vi "Mouse Init.vi"(2 "Timeout (ms)":i32=100, 3 "FPGA VI Reference In":refnum<k20>) -> (0 "Timed out?":bool, 1 "Mouse Sensor":T1)   [LabVIEW 2012, in "Mouse IO.lvlib"]
uses:
  Mouse IO.lvlib
panel:
  # "Mouse Interface\n===\nInitialise and begin Mouse Sensor.\nReturns Mouse Sensor cluster to pass to Mouse Loop.vi\nTimeout in 100's of milliseconds."
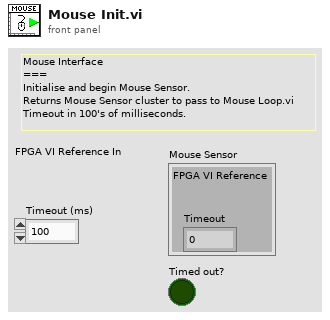
[diagram p1: front panel]
types:
  T1 = cluster{"FPGA VI Reference":refnum<k20>, "Timeout":i32}
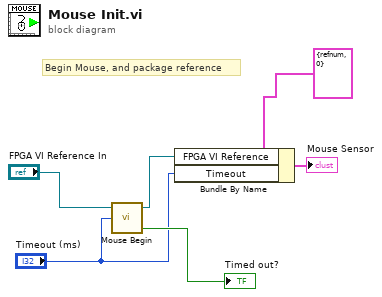
[diagram p0: block diagram]
diagram:
  # "Begin Mouse, and package reference"
  n1 = call "Mouse Begin.vi"("Timeout (ms)"="Timeout (ms)", "FPGA VI Reference In"="FPGA VI Reference In") -> ("Timed out?"=→"Timed out?":bool, "FPGA VI Reference Out"=w3:refnum<k20>)  [unwired: 2 in]
  n2 = Bundle By Name(cluster=T1 {"FPGA VI Reference"=refnum, "Timeout"=0} ("Mouse Sensor"), "FPGA VI Reference"=w3, "Timeout"="Timeout (ms)") -> (→"Mouse Sensor":T1)
